vi "1CellLog.vi"(1 "CellV":dbl) -> ()   [LabVIEW 2025]
uses:
  <vilib>/httpClient/LabVIEWHTTPClient.lvlib
panel:
  out "body":string
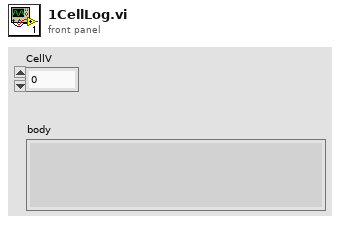
[diagram p1: front panel]
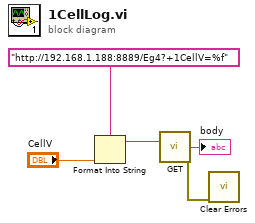
[diagram p0: block diagram]
diagram:
  n1 = Format Into String(format string="http://192.168.1.188:8889/Eg4?+1CellV=%f", "CellV") -> (resulting string=w2:string)  [unwired: 2 in, 1 out]
  n2 = call <vilib>:"GET.vi"("url"=w2) -> ("body"=→"body":string, "error out"=w4:errorcluster)  [unwired: 11 in, 2 out]
  n3 = call <vilib>:"Clear Errors.vi"("error in (no error)"=w4) -> ()  [unwired: 5 in, 2 out]
